vi "Reaction_Game.vi"() -> ()   [LabVIEW 2017]
panel:
  in  "stop":bool
  out "Result":dbl
  out "Message":string
  in  "PushButton":bool
  out "Indicator":bool
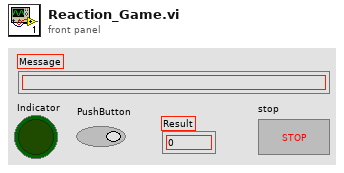
[diagram p1: front panel]
types:
  T1 = enum16{"Hello", "RandomWait", "WaitForClick", "Calculate"}
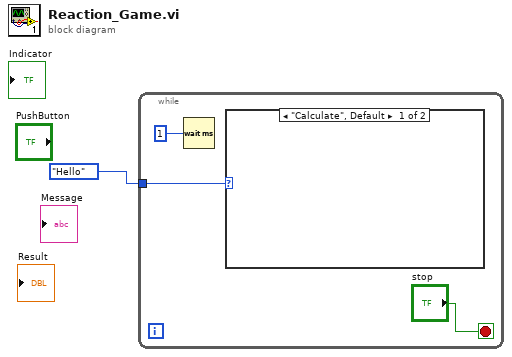
[diagram p0: block diagram]
diagram:
  n1 = while {
    tunnel: T1."Hello" -> [w2]
    stop <- "stop" stop-if-true
    n2 = Wait (ms)(milliseconds to wait=1) -> ()  [unwired: 1 out]
    n3 = case shown="\"Calculate\", Default" w2 {
      frame "Calculate", Default {
      }
      frame "WaitForClick" {
      }
    }
  }
